vi "FPGA-conrol_of Tank1.vi"() -> ()   [LabVIEW 2012]
uses:
  <vilib>/rvi/eio/common/nirviEmuTemplateMethod_errors.vi
  <vilib>/eio/EIONode/EIONode.xnode
panel:
  in  "stop":bool
  in  "Port9/DIO8":bool
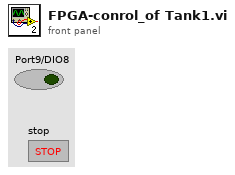
[diagram p1: front panel]
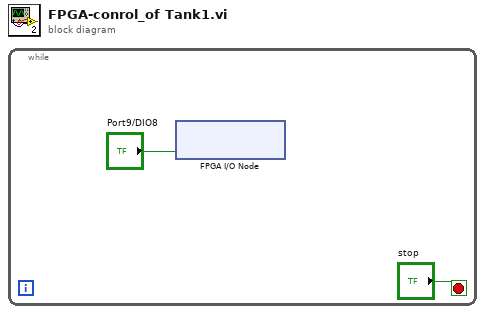
[diagram p0: block diagram]
diagram:
  n1 = while {
    stop <- "stop" stop-if-true
    n2 = xnode "FPGA I/O Node"("Port9/DIO8"="Port9/DIO8") -> ()  [unwired: 1 in, 1 out]
  }
